vi "Rearrange Into 1D Array.vi"(8 "Error In":errorcluster, 10 "RGB Gains":T1, 11 "Matrix":u32[][](array[colorbox])) -> (0 "Error Out":errorcluster, 3 "Raw Data":u8[](array[numeric]))   [LabVIEW 2021, in "Display.lvclass"]
uses:
  Display.lvclass
  Public/Controls/RGB Gains.ctl
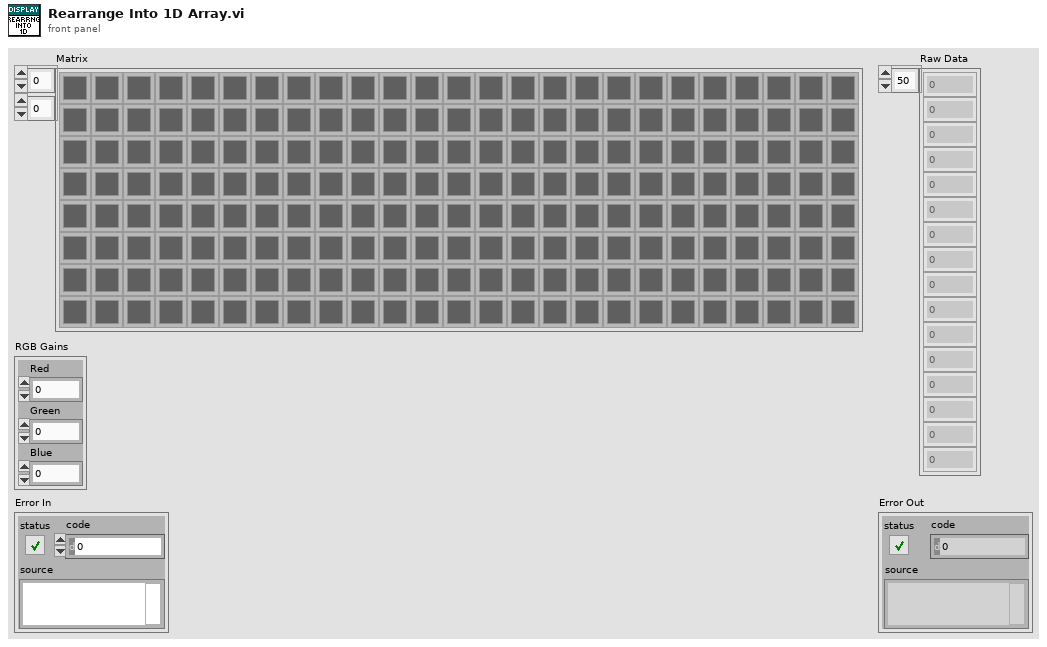
[diagram p1: front panel]
types:
  T1 = typedef "Display.lvclass/RGB Gains.ctl" = cluster{"Red":sgl, "Green":sgl, "Blue":sgl}
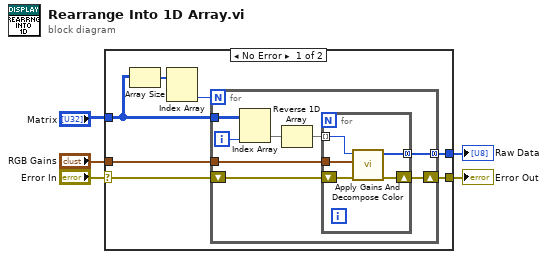
[diagram p0: block diagram]
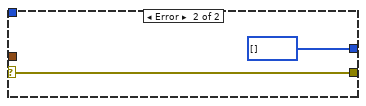
[diagram p2: hidden frame]
diagram:
  n1 = case shown="No Error" "Error In" {
    selector: "Error In" -> [w8 w27]
    tunnel: [w6 u8[] []] -> w5
    tunnel: "RGB Gains" -> [w9 _]
    tunnel: "Matrix" -> [w11 _]
    tunnel: [w7 w27] -> w1
    frame No Error {
      n2 = Array Size(array=w11) -> (size(s)=w12:i32[])
      n3 = Index Array(array=w12) -> (element #2=w10:i32)  [unwired: 2 in, 1 out]
      n4 = for {
        N: w10 -> [_]
        tunnel: w11 -> [w20]
        tunnel: w9 -> [w18]
        shift-right: [w16] -> w7
        shift-left: w8 -> [w17]
        tunnel: [w13] -> w6 mode=concatenating
        i -> [w15]
        n5 = Index Array(array=w20, index (col)=w15) -> (element=w14:u32[])  [unwired: 1 in]
        n6 = Reverse 1D Array(array=w14) -> (reversed array=w19:u32[])
        n7 = for {
          tunnel: w19 -> [w25] mode=indexing
          tunnel: w18 -> [w24]
          shift-right: [w22] -> w16
          shift-left: w17 -> [w23]
          tunnel: [w21] -> w13 mode=concatenating
          n8 = call "Apply Gains And Decompose Color.vi"("Error In"=w23, "RGB Gains"=w24, "Color Box"=w25) -> ("Error Out"=w22:errorcluster, "Data"=w21:u8[])  [unwired: 7 in]
        }
      }
    }
    frame Error {
    }
  }
  "Raw Data" <- w5
  "Error Out" <- w1
